vi "Returning A Value Simple Struct Added.vi"(8 "error in (no error)":errorcluster) -> (0 "error out":errorcluster, 3 "function return":i32)   [LabVIEW 2009, in "LabVIEWWrapper_PassingDataSampleDLL.lvlib"]
doc: "int ReturningAValue_Integer (void);"
uses:
  LabVIEWWrapper_PassingDataSampleDLL.lvlib
  CustomControlsForStructs/SimpleStruct Circle.ctl
  <vilib>/Utility/importsl/GetValueByPointer/GetValueByPointer.xnode
  <vilib>/Utility/importsl/GetValueByPointer/datatype.ctl
  Program Files (x86)/National Instruments/LabVIEW 2009/resource/lvimptsl.dll
  PassingDataSampleDLL.dll
panel:
  out "Output":T1
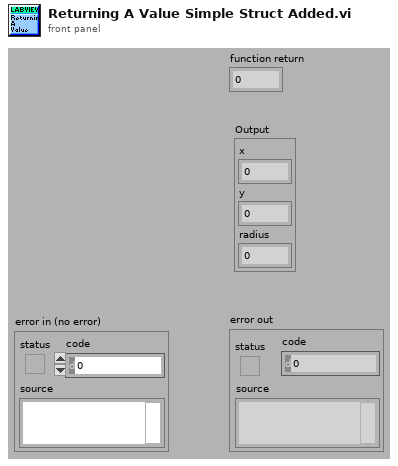
[diagram p1: front panel]
types:
  T1 = typedef "LabVIEWWrapper_PassingDataSampleDLL.lvlib/SimpleStruct Circle.ctl" = cluster{"x":sgl, "y":sgl, "radius":sgl}
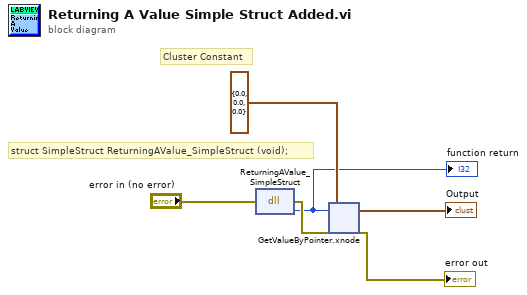
[diagram p0: block diagram]
diagram:
  # "Cluster Constant"
  # "struct SimpleStruct ReturningAValue_SimpleStruct (void);"
  n1 = dll-call lib="C:/My Dropbox/Partner Program/SDK/Calling External Code/Example Calling C_C++ DLLs Containing Simple and Complex Datatypes from LabVIEW/Files/LabVIEWWrapper/PassingDataSampleDLL.*" fn="ReturningAValue_SimpleStruct"(error in="error in (no error)") -> (error out=w3:errorcluster, "return type"=w1:i64)  [unwired: 2 in, 1 out]
  "function return" <- w1
  n2 = xnode "GetValueByPointer.xnode"("Pointer"=w1, "InputType"=cluster{"x":sgl, "y":sgl, "radius":sgl} {"x"=0.0, "y"=0.0, "radius"=0.0} ("Circle"), "ErrorIn"=w3) -> ("Output"=→"Output":cluster{"x":sgl, "y":sgl, "radius":sgl}, "ErrorOut"=→"error out":errorcluster)  [unwired: 1 in]
